vi "De-Indent.vi"(11 "MsgSerializer in":refnum<class "MsgSerializer.lvclass">) -> (3 "MsgSerializer out":refnum<class "MsgSerializer.lvclass">)   [LabVIEW 2013, in "Caraya.lvlib" / "MsgSerializer.lvclass"]
uses:
  MsgSerializer.lvclass
  MsgSerializer.lvclass/MsgSerializer.ctl
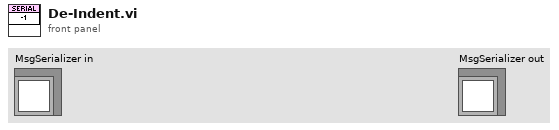
[diagram p1: front panel]
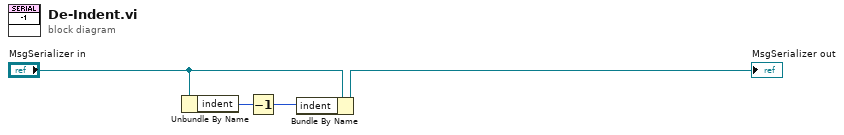
[diagram p0: block diagram]
diagram:
  n1 = Unbundle By Name("MsgSerializer in") -> ("indent"=w4:i32)
  n2 = Decrement(x=w4) -> (x-1=w3:i32)
  n3 = Bundle By Name(cluster="MsgSerializer in", "indent"=w3) -> (→"MsgSerializer out":refnum<class "MsgSerializer.lvclass">)
